vi "Channel Data and Porperties to Table.vi"(8 "error in (no error)":errorcluster, 11 "Node Ptr":T1 format="%.0x") -> (0 "error out":errorcluster, 2 "Properties List Out":string[][](array[string]), 3 "Channel Ref out":T1 format="%.0x")   [LabVIEW 2017, in "Scan Engine Custom Device.lvlib"]
uses:
  Scan Engine Custom Device.lvlib
  <vilib>/NI Veristand/Custom Device API/Custom Device Item Ref.ctl
  <vilib>/NI VeriStand/Custom Device API/Custom Device API.lvlib
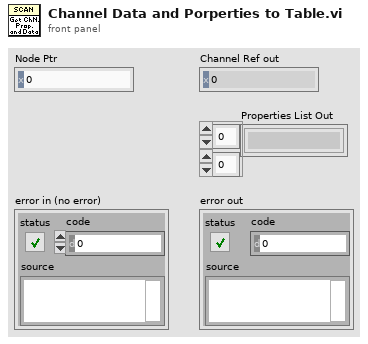
[diagram p1: front panel]
types:
  T1 = typedef "Custom Device API.lvlib/Custom Device Item Ref.ctl" = u64
  T2 = typedef "Custom Device API.lvlib/Custom Device Channel.ctl" = cluster{"Type":T3, "Units":string, "Default Value":dbl, "Faultable":bool, "Scalable":bool}
  T3 = typedef "Custom Device API.lvlib/Custom Device Channel Type.ctl" = enum16{"Input", "Output"}
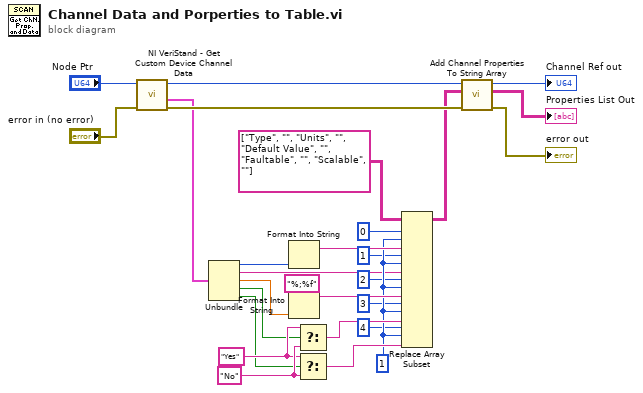
[diagram p0: block diagram]
diagram:
  w18 = "No"
  w17 = "Yes"
  w13 = 1 ("disabled index (col)")
  n1 = call <vilib>:"NI VeriStand - Get Custom Device Channel Data.vi"("error in (no error)"="error in (no error)", "Channel Ref in"="Node Ptr") -> ("error out"=w24:errorcluster, "Channel"=w8:T2, "Channel Ref out"=w1:T1)  [unwired: 4 in, 3 out]
  n2 = Unbundle(w8) -> ("Type"=w3:T3, "Units"=w7:string, "Default Value"=w4:dbl, "Faultable"=w5:bool, "Scalable"=w6:bool)
  n3 = Format Into String(w3) -> (resulting string=w19:string)  [unwired: 3 in, 1 out]
  n4 = Format Into String(format string="%;%f", w4) -> (resulting string=w20:string)  [unwired: 2 in, 1 out]
  n5 = Select(t=w17, s=w5, f=w18) -> (s? t:f=w21:string)
  n6 = Select(t=w17, s=w6, f=w18) -> (s? t:f=w22:string)
  n7 = Replace Array Subset(array=string[][] [["Type", ""], ["Units", ""], ["Default Value", ""], ["Faultable", ""], ["Scalable", ""]], new element #1=w19, index (row) #1=0 ("disabled index (row)"), index (col) #1=w13, new element #2=w7, index (row) #2=1 ("disabled index (row)"), index (col) #2=w13, new element #3=w20, index (row) #3=2 ("disabled index (row)"), index (col) #3=w13, new element #4=w21, index (row) #4=3 ("disabled index (row)"), index (col) #4=w13, new element #5=w22, index (row) #5=4 ("disabled index (row)"), index (col) #5=w13) -> (w2:string[][])
  n8 = call "Add Channel Properties To String Array.vi"("error in"=w24, "Properties List In"=w2, "Channel Ref in"=w1) -> ("error out"=→"error out":errorcluster, "Properties List Out"=→"Properties List Out":string[][], "Channel Ref out"=→"Channel Ref out":T1)  [unwired: 6 in]
